vi "AprilTag_Equals.vi"(9 "Other AprilTag":T1={"ID"=0, "POSE3D"={"Translation3d"={"X"=0.0, "Y"=0.0, "Z"=0.0}, "Rotation3d"={"Q_quaternion"={"R"=1.0, "V"=[0.0, 0.0, 0.0]}}}} {"POSE3D"."Translation3d"."Z" format="%14.3f"; "POSE3D"."Translation3d"."Y" format="%14.3f"; "POSE3D"."Translation3d"."X" format="%14.3f"}, 11 "AprilTag":T1={"ID"=0, "POSE3D"={"Translation3d"={"X"=0.0, "Y"=0.0, "Z"=0.0}, "Rotation3d"={"Q_quaternion"={"R"=1.0, "V"=[0.0, 0.0, 0.0]}}}} {"POSE3D"."Translation3d"."Z" format="%14.3f"; "POSE3D"."Translation3d"."Y" format="%14.3f"; "POSE3D"."Translation3d"."X" format="%14.3f"}) -> (3 "Equal":bool)   [LabVIEW 2019, in "Trajectory_Library.lvlib"]
doc: "Determine if two April Tag data clusters are equal.\n\nInputs:\n -- AprilTag -- AprilTag -- First data cluster to check\n -- OtherAprilTag -- AprilTag -- Second data cluster to check\n\nOutputs:\n -- Equal -- Boolean -- TRUE if both data clusters are the same."
uses:
  Trajectory_Library.lvlib
  TypeDef/AprilTag.ctl
  TypeDef/POSE3D.ctl
  TypeDef/TRANSLATION3D.ctl
  TypeDef/ROTATION3D.ctl
  TypeDef/QUATERNION.ctl
  Translation3d_Equals.vi
  Rotation3d_Equals.vi
  Pose3d_getTranslation3d.vi
  Pose3d_getRotation3d.vi
  Rotation3d_GetQuaterion.vi
  Quaternion_Equals.vi
  Quaternion_Get_Vect.vi
  Quaternion_Get_W.vi
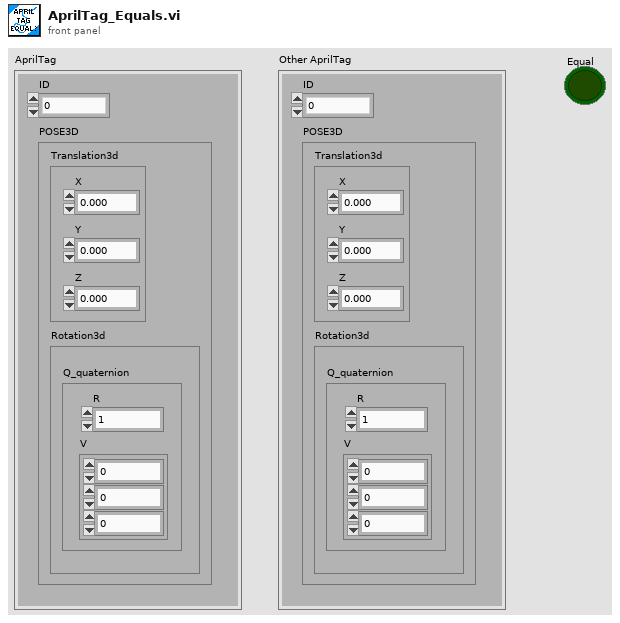
[diagram p1: front panel]
types:
  T1 = typedef "Trajectory_Library.lvlib/AprilTag.ctl" = cluster{"ID":i32, "POSE3D":T2}
  T2 = typedef "Trajectory_Library.lvlib/POSE3D.ctl" = cluster{"Translation3d":T3, "Rotation3d":T4}
  T3 = typedef "Trajectory_Library.lvlib/TRANSLATION3D.ctl" = cluster{"X":dbl, "Y":dbl, "Z":dbl}
  T4 = typedef "Trajectory_Library.lvlib/ROTATION3D.ctl" = cluster{"Q_quaternion":T5}
  T5 = typedef "Trajectory_Library.lvlib/QUATERNION.ctl" = cluster{"R":dbl, "V":dbl[]}
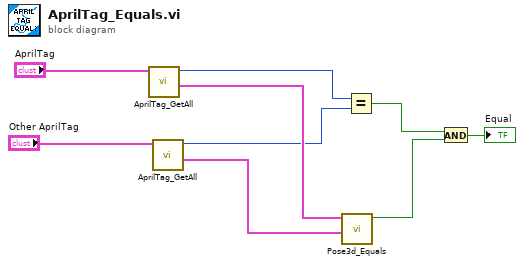
[diagram p0: block diagram]
diagram:
  n1 = call "AprilTag_GetAll.vi"("AprilTag"="AprilTag") -> ("POSE3D"=w7:T2, "ID"=w5:i32)  [unwired: 9 in]
  n2 = call "AprilTag_GetAll.vi"("AprilTag"="Other AprilTag") -> ("POSE3D"=w6:T2, "ID"=w4:i32)  [unwired: 9 in]
  n3 = call "Pose3d_Equals.vi"("other Pose3d"=w6, "in Pose3d"=w7) -> ("Equals"=w2:bool)  [unwired: 9 in]
  n4 = Equal?(x=w5, y=w4) -> (x = y?=w3:bool)
  n5 = And(x=w3, y=w2) -> (x .and. y?=→"Equal":bool)
